vi "macro_NumCmd_Send_Chassis.vi"() -> ()   [LabVIEW 2019, in "Trajectory_Library.lvlib"]
uses:
  VI/numCmd_Recv_Generic.vi
  VI/numCmd_ObtainQueue_Generic.vi
  Trajectory_Library.lvlib
  TypeDef/CHASSIS_SPEEDS.ctl
panel:
  in  "SwerveSpeedDemand":T1 {"vOmega" format="%10.3f"; "vY" format="%10.3f"; "vX" format="%10.3f"}
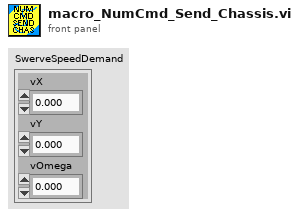
[diagram p1: front panel]
types:
  T1 = typedef "Trajectory_Library.lvlib/CHASSIS_SPEEDS.ctl" = cluster{"vX":dbl, "vY":dbl, "vOmega":dbl}
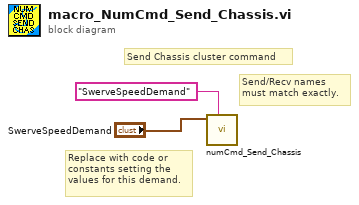
[diagram p0: block diagram]
diagram:
  # "Replace with code or\nconstants setting the \nvalues for this demand."
  # "Send/Recv names\nmust match exactly."
  # "Send Chassis cluster command"
  n1 = call "numCmd_Send_Chassis.vi"("Command Name"="SwerveSpeedDemand", "Chassis Speeds"="SwerveSpeedDemand") -> ()  [unwired: 9 in, 1 out]
